vi "DrawAttributes.vi"(1 "Parameters":T2, 2 "rect":cluster{sgl, sgl, sgl, sgl}, 3 "upper Left":cluster{sgl, sgl}, 4 "image in":picture) -> (0 "image out":picture)   [LabVIEW 2014]
uses:
  ParamterCluster.ctl
panel:
  in  "[user-specified font]":T1={"Font Name:"="Verdana", "Size"=32, "Strikeout?"=FALSE, "Italic?"=FALSE, "Underline?"=FALSE, "Outline?"=FALSE, "Shadow?"=FALSE, "Bold?"=FALSE}
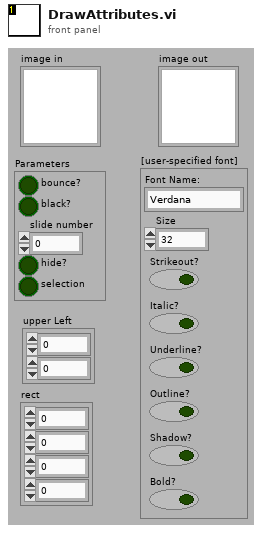
[diagram p1: front panel]
types:
  T1 = cluster{"Font Name:":string, "Size":i16, "Strikeout?":bool, "Italic?":bool, "Underline?":bool, "Outline?":bool, "Shadow?":bool, "Bold?":bool}
  T2 = typedef "ParamterCluster.ctl" = cluster{"bounce?":bool, "black?":bool, "slide number":i32, "hide?":bool, "selection":bool}
  T3 = enum16{"User-specified Font", "Application Font", "System Font", "Dialog Font"}
  T4 = cluster{"Width":i16, "Style":enum32{"Solid", "Dash", "Dot", "DashDot", "DashDotDot"}}
  T5 = cluster{"left":i16, "top":i16, "right":i16, "bottom":i16}
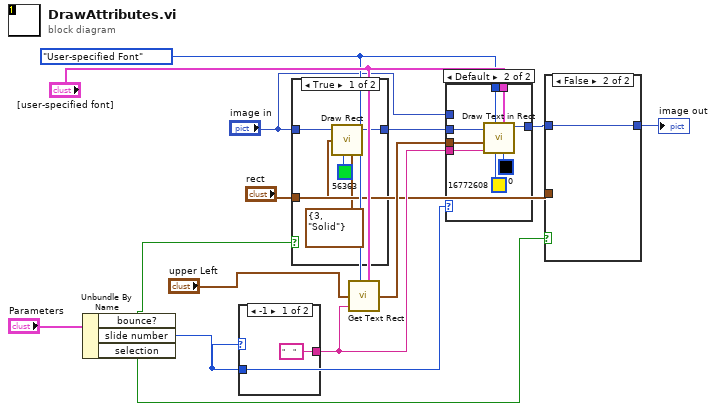
[diagram p0: block diagram]
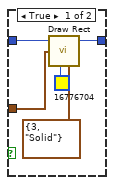
[diagram p2: hidden frame]
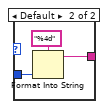
[diagram p4: hidden frame]
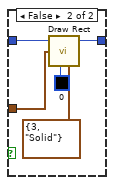
[diagram p5: hidden frame]
diagram:
  w7 = T3."User-specified Font" ("desired font(Application)")
  n1 = Unbundle By Name("Parameters") -> ("bounce?"=w10:bool, "slide number"=w5:i32, "selection"=w1:bool)
  n2 = case shown="-1" w5 {
    tunnel: ["    " w18] -> w12
    tunnel: w5 -> [_ w16]
    frame -1 {
    }
    frame Default {
      n3 = Format Into String(format string="%4d", w16) -> (resulting string=w18:string)  [unwired: 2 in, 1 out]
    }
  }
  n4 = case shown="True" w10 {
    tunnel: "image in" -> [w23 w28]
    tunnel: [w22 w27] -> w11
    tunnel: "rect" -> [w21 w26]
    frame True {
      n5 = call <vilib>:"Draw Rect.vi"("picture"=w23, "rect"=w21, "color(black)"=u32 56363, "pen"=T4 {"Width"=3, "Style"=enum."Solid"}) -> ("new picture"=w22:picture)  [unwired: 5 in]
    }
    frame False {
      n6 = call <vilib>:"Draw Rect.vi"("picture"=w28, "rect"=w26, "color(black)"=u32 0, "pen"=T4 {"Width"=3, "Style"=enum."Solid"}) -> ("new picture"=w27:picture)  [unwired: 5 in]
    }
  }
  n7 = call <vilib>:"Get Text Rect.vi"("desired font(Application)"=w7, "origin(0,0)"="upper Left", "text"=w12, "[user-specified font]"="[user-specified font]") -> ("rect"=w14:T5)  [unwired: 5 in]
  n8 = case shown="Default" w5 {
    tunnel: w14 -> [_ w37]
    tunnel: w12 -> [_ w36]
    tunnel: [w29 w34] -> w4
    tunnel: w11 -> [w29 w32]
    tunnel: "[user-specified font]" -> [_ w31]
    tunnel: w7 -> [_ w30]
    tunnel: "image in" -> [_ _]
    frame -1 {
    }
    frame Default {
      n9 = call <vilib>:"Draw Text in Rect.vi"("BG color(transparent)"=u32 0, "[user-specified font]"=w31, "text color(black)"=u32 16772608, "desired font(Application)"=w30, "text"=w36, "rect"=w37, "picture"=w32) -> ("new picture"=w34:picture)  [unwired: 4 in]
    }
  }
  n10 = case shown="False" w1 {
    tunnel: w4 -> [w42 w43]
    tunnel: [w41 w43] -> w3
    tunnel: "rect" -> [w40 _]
    frame True {
      n11 = call <vilib>:"Draw Rect.vi"("picture"=w42, "rect"=w40, "color(black)"=u32 16776704, "pen"=T4 {"Width"=3, "Style"=enum."Solid"}) -> ("new picture"=w41:picture)  [unwired: 5 in]
    }
    frame False {
    }
  }
  "image out" <- w3
